vi "Agilent SNA Read IFBW.vi"(6 "Channel":i8=1 min=1 max=99 step=1, 7 "Agilent SNA & SWP":T2, 8 "error in (no error)":errorcluster, 11 "VISA Resource Names":T1) -> (0 "error out":errorcluster, 2 "IFBW, Hz":dbl=3000.0, 3 "dup VISA Resource Name":T1)   [LabVIEW 2011]
doc: "This Vi for the HP8753B Network Analyzer is used to set averaging, smoothing, and the IF bandwidth."
uses:
  TypeDefs/Agilent SNA VISA.ctl
  TypeDefs/Agilent SNA Instrument Info.ctl
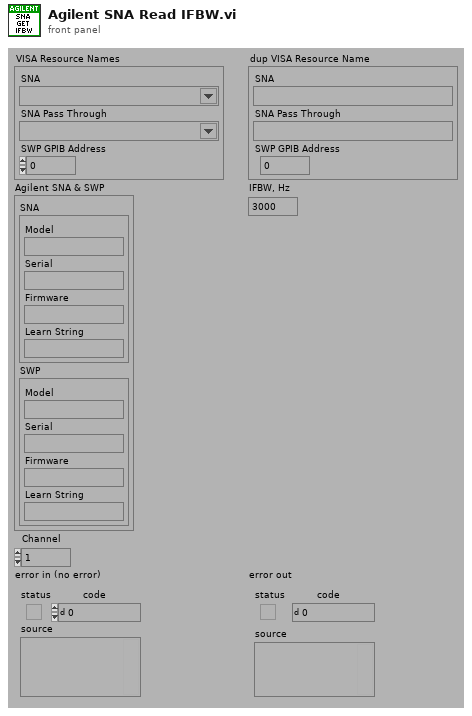
[diagram p1: front panel]
types:
  T1 = typedef "Agilent SNA VISA.ctl" = cluster{"SNA":refnum<visa-resource-name>, "SNA Pass Through":refnum<visa-resource-name>, "SWP GPIB Address":i32}
  T2 = typedef "Agilent SNA Instrument Info.ctl" = cluster{"SNA":cluster{"Model":string, "Serial":string, "Firmware":string, "Learn String":string}, "SWP":cluster{"Model":string, "Serial":string, "Firmware":string, "Learn String":string}}
  T3 = typedef "Agilent SNA Model.ctl" = enum16{"Not Supported", "8757X"}
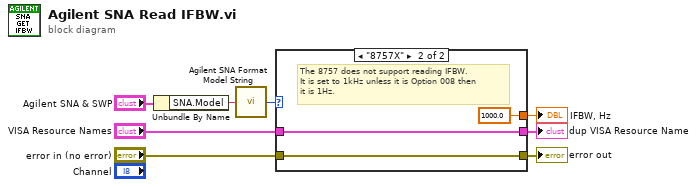
[diagram p0: block diagram]
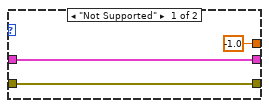
[diagram p2: hidden frame]
diagram:
  n1 = Unbundle By Name("Agilent SNA & SWP") -> ("SNA.Model"=w1:string)
  n2 = call "Agilent SNA Format Model String.vi"("Model String"=w1) -> ("Model"=w3:T3)
  n3 = case shown="\"8757X\"" w3 {
    tunnel: "VISA Resource Names" -> [w10 w13]
    tunnel: "error in (no error)" -> [w11 w14]
    tunnel: [w10 w13] -> w6
    tunnel: [w11 w14] -> w5
    tunnel: [-1.0 1000.0] -> w4
    frame "Not Supported" {
    }
    frame "8757X" {
      # "The 8757 does not support reading IFBW.\nIt is set to 1kHz unless it is Option 008 then\nit is 1Hz."
    }
  }
  "error out" <- w5
  "dup VISA Resource Name" <- w6
  "IFBW, Hz" <- w4
